vi "ConfigureIntake.vi"(10 "Talon In":T1) -> (2 "Talon Out":T1)   [LabVIEW 2018]
uses:
  <vilib>/Rock Robotics/WPI/MotorControl/WPI_MotorControlDeviceRef.ctl
  <vilib>/Rock Robotics/WPI/MotorControl/WPI_MotorControlType.ctl
  <vilib>/Rock Robotics/SystemInterfaces/DIO/FPGA_DIOPWMChannel.ctl
  <vilib>/Rock Robotics/WPI/PWM/WPI_PWMDeadband.ctl
  <vilib>/Rock Robotics/SystemInterfaces/DIO/FPGA_DIOChannel.ctl
  <vilib>/Rock Robotics/WPI/ThirdParty/Phoenix-LabVIEW/Motor Controller/Controls/CTRE_Phoenix_MotorControl_FeedbackDevice.ctl
  <vilib>/Rock Robotics/WPI/ThirdParty/Phoenix-LabVIEW/Motor Controller/Controls/CTRE_Phoenix_MotorControl_StatusFrameEnhanced.ctl
  <vilib>/Rock Robotics/WPI/ThirdParty/Phoenix-LabVIEW/Motor Controller/Controls/CTRE_Phoenix_MotorControl_NeutralMode.ctl
  <vilib>/Rock Robotics/WPI/ThirdParty/Phoenix-LabVIEW/Motor Controller/Controls/CTRE_Phoenix_MotorControl_ControlMode.ctl
  Intake Constants.vi
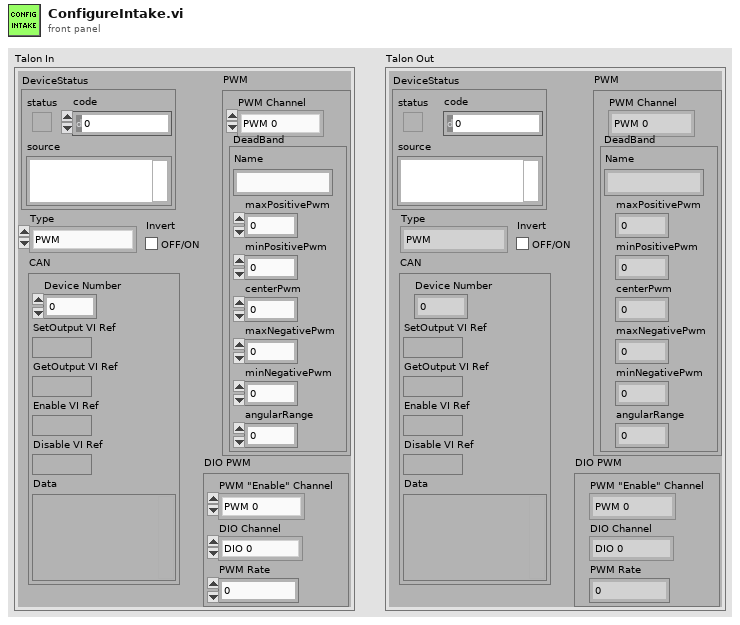
[diagram p1: front panel]
types:
  T1 = typedef "WPI_MotorControlDeviceRef.ctl" = cluster{"DeviceStatus":errorcluster, "Type":T2, "PWM":cluster{"PWM Channel":T3, "DeadBand":T4}, "CAN":cluster{"Device Number":u8, "SetOutput VI Ref":variant, "GetOutput VI Ref":variant, "Enable VI Ref":variant, "Disable VI Ref":variant, "Data":variant}, "Invert":bool, "DIO PWM":cluster{"PWM \"Enable\" Channel":T3, "DIOChannel":T5, "PWM Rate":dbl}}
  T2 = typedef "WPI_MotorControlType.ctl" = enum16{"PWM", "CAN", "DIO PWM"}
  T3 = typedef "FPGA_DIOPWMChannel.ctl" = enum8{"PWM 0", "PWM 1", "PWM 2", "PWM 3", "PWM 4", "PWM 5", "PWM 6", "PWM 7", "PWM 8", "PWM 9", "PWM MXP 0", "PWM MXP 1", "PWM MXP 2", "PWM MXP 3", "PWM MXP 4", "PWM MXP 5", "PWM MXP 6", "PWM MXP 7", "PWM MXP 8", "PWM MXP 9", "Invalid"}
  T4 = typedef "WPI_PWMDeadband.ctl" = cluster{"Name":string, "maxPositivePwm":i32, "minPositivePwm":i32, "centerPwm":i32, "maxNegativePwm":i32, "minNegativePwm":i32, "angularRange":u16}
  T5 = typedef "FPGA_DIOChannel.ctl" = enum8{"DIO 0", "DIO 1", "DIO 2", "DIO 3", "DIO 4", "DIO 5", "DIO 6", "DIO 7", "DIO 8", "DIO 9", "DIO MXP 0", "DIO MXP 1", "DIO MXP 2", "DIO MXP 3", "DIO MXP 4", "DIO MXP 5", "DIO MXP 6", "DIO MXP 7", "DIO MXP 8", "DIO MXP 9", "DIO MXP 10", "DIO MXP 11", "DIO MXP 12", "DIO MXP 13", "DIO MXP 14", "DIO MXP 15", "SPI Port CS1", "SPI Port CS2", "SPI Port CS3", "SPI Port MISO", "SPI Port MOSI", "Invalid"}
  T6 = typedef "CTRE_Phoenix_MotorControl_ControlMode.ctl" = u16
  T7 = typedef "CTRE_Phoenix_MotorControl_NeutralMode.ctl" = enum8{"EEPROMSetting", "Override to Coast", "Override to Brake"}
  T8 = typedef "CTRE_Phoenix_MotorControl_StatusFrameEnhanced.ctl" = u16
  T9 = typedef "CTRE_Phoenix_MotorControl_FeedbackDevice.ctl" = i8
  T10 = cluster{"kP":dbl, "kI ":dbl, "kD":dbl, "kF":dbl, "I Zone":dbl, "Peak Out":dbl}
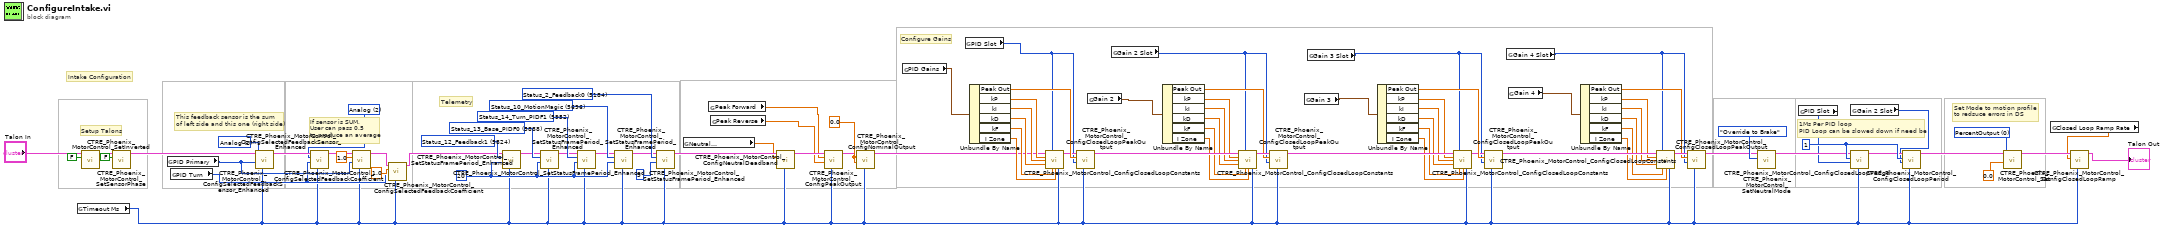
[diagram p0: block diagram]
diagram:
  w29 = T6 0 items=["PercentOutput"=0, "Position"=1, "Velocity"=2, "Current"=3, "Follower"=5, "MotionProfile"=6, "MotionMagic"=7, "MotionProfileArc"=10, "Disabled"=15] ("Control Mode")
  w87 = 1 ("loopTimeMs")
  w50 = 0.0 ("Forward Nominal Percent Output")
  w26 = 20 ("periodMs")
  w45 = T8 5184 items=["Status_1_General"=5120, "Status_2_Feedback0"=5184, "Status_3_Quadrature"=5248, "Status_4_AinTempVbat"=5312, "Status_6_Misc"=5440, "Status_7_CommStatus"=5504, "Status_8_PulseWidth"=5568, "Status_9_MotProfBuffer"=5632, "Status_10_MotionMagic"=5696, "Status_11_UartGadgeteer"=5760, "Status_12_Feedback1"=5824, "Status_13_Base_PIDF0"=5888, "Status_14_Turn_PIDF1"=5952, "Status_15_FirmwareApiStatus"=6016] ("Status Frame")
  w44 = T8 5696 items=["Status_1_General"=5120, "Status_2_Feedback0"=5184, "Status_3_Quadrature"=5248, "Status_4_AinTempVbat"=5312, "Status_6_Misc"=5440, "Status_7_CommStatus"=5504, "Status_8_PulseWidth"=5568, "Status_9_MotProfBuffer"=5632, "Status_10_MotionMagic"=5696, "Status_11_UartGadgeteer"=5760, "Status_12_Feedback1"=5824, "Status_13_Base_PIDF0"=5888, "Status_14_Turn_PIDF1"=5952, "Status_15_FirmwareApiStatus"=6016] ("Status Frame")
  w43 = T8 5952 items=["Status_1_General"=5120, "Status_2_Feedback0"=5184, "Status_3_Quadrature"=5248, "Status_4_AinTempVbat"=5312, "Status_6_Misc"=5440, "Status_7_CommStatus"=5504, "Status_8_PulseWidth"=5568, "Status_9_MotProfBuffer"=5632, "Status_10_MotionMagic"=5696, "Status_11_UartGadgeteer"=5760, "Status_12_Feedback1"=5824, "Status_13_Base_PIDF0"=5888, "Status_14_Turn_PIDF1"=5952, "Status_15_FirmwareApiStatus"=6016] ("Status Frame")
  w42 = T8 5888 items=["Status_1_General"=5120, "Status_2_Feedback0"=5184, "Status_3_Quadrature"=5248, "Status_4_AinTempVbat"=5312, "Status_6_Misc"=5440, "Status_7_CommStatus"=5504, "Status_8_PulseWidth"=5568, "Status_9_MotProfBuffer"=5632, "Status_10_MotionMagic"=5696, "Status_11_UartGadgeteer"=5760, "Status_12_Feedback1"=5824, "Status_13_Base_PIDF0"=5888, "Status_14_Turn_PIDF1"=5952, "Status_15_FirmwareApiStatus"=6016] ("Status Frame")
  w41 = T8 5824 items=["Status_1_General"=5120, "Status_2_Feedback0"=5184, "Status_3_Quadrature"=5248, "Status_4_AinTempVbat"=5312, "Status_6_Misc"=5440, "Status_7_CommStatus"=5504, "Status_8_PulseWidth"=5568, "Status_9_MotProfBuffer"=5632, "Status_10_MotionMagic"=5696, "Status_11_UartGadgeteer"=5760, "Status_12_Feedback1"=5824, "Status_13_Base_PIDF0"=5888, "Status_14_Turn_PIDF1"=5952, "Status_15_FirmwareApiStatus"=6016] ("Status Frame")
  w25 = T9 2 items=["None"=-1, "QuadEncoder"=0, "Analog"=2, "Tachometer"=4, "Pulse Width Encoded Position"=8, "Sensor Sum (S0 + S1)"=9, "Sensor Difference (D0 - D1)"=10, "Remote Source 0"=11, "Remote Source 1"=12, "Software Emulated"=15] ("Feedback Device")
  w33 = T9 2 items=["None"=-1, "QuadEncoder"=0, "Analog"=2, "Tachometer"=4, "Pulse Width Encoded Position"=8, "Sensor Sum (S0 + S1)"=9, "Sensor Difference (D0 - D1)"=10, "Remote Source 0"=11, "Remote Source 1"=12, "Software Emulated"=15] ("Feedback Device")
  # "Intake Configuration"
  # "Set Mode to motion profile\nto redsuce errors in DS"
  # "1Ms Per PID loop\nPID Loop can be slowed down if need be"
  # "Configure Gains"
  # "Setup Talons"
  # "Telemetry"
  # "If sensor is SUM,\nUser can pass 0.5\nto produce an average"
  # "This feedback sensor is the sum\nof left side and this one (right side)"
  n1 = global read "Intake Constants.vi" "Timeout Ms"() -> (w2:i32)
  n2 = call <vilib>:"CTRE_Phoenix_MotorControl_SetInverted.vi"("Invert?"=FALSE, "PhoenixMotorControlDevRef"="Talon In") -> ("PhoenixMotorControlDevRef"=w31:T1)  [unwired: 8 in, 1 out]
  n3 = call <vilib>:"CTRE_Phoenix_MotorControl_SetSensorPhase.vi"("PhaseSensor"=FALSE, "PhoenixMotorControlDevRef"=w31) -> ("PhoenixMotorControlDevRef"=w22:T1)  [unwired: 8 in, 1 out]
  n4 = global read "Intake Constants.vi" "PID Primary"() -> (w19:i32)
  n5 = global read "Intake Constants.vi" "PID Turn"() -> (w18:i32)
  n6 = call <vilib>:"CTRE_Phoenix_MotorControl_ConfigSelectedFeedbackSensor_Enhanced.vi"("timeoutMs"=w2, "pidLoopIdx"=w19, "Feedback Device"=w33, "PhoenixMotorControlDevRef"=w22) -> ("PhoenixMotorControlDevRef"=w34:T1)  [unwired: 6 in, 1 out]
  n7 = call <vilib>:"CTRE_Phoenix_MotorControl_ConfigSelectedFeedbackSensor_Enhanced.vi"("timeoutMs"=w2, "pidLoopIdx"=w18, "Feedback Device"=w25, "PhoenixMotorControlDevRef"=w34) -> ("PhoenixMotorControlDevRef"=w35:T1)  [unwired: 6 in, 1 out]
  n8 = call <vilib>:"CTRE_Phoenix_MotorControl_ConfigSelectedFeedbackCoefficient.vi"("timoutMs"=w2, "pidIdx"=w19, "coefficient"=1.0, "PhoenixMotorControlDevRef"=w35) -> ("PhoenixMotorControlDevRef"=w24:T1)  [unwired: 6 in, 1 out]
  n9 = call <vilib>:"CTRE_Phoenix_MotorControl_ConfigSelectedFeedbackCoefficient.vi"("timoutMs"=w2, "pidIdx"=w18, "coefficient"=1.0, "PhoenixMotorControlDevRef"=w24) -> ("PhoenixMotorControlDevRef"=w23:T1)  [unwired: 6 in, 1 out]
  n10 = call <vilib>:"CTRE_Phoenix_MotorControl_SetStatusFramePeriod_Enhanced.vi"("timeoutMs"=w2, "periodMs"=w26, "Status Frame"=w41, "PhoenixMotorControlDevRef"=w23) -> ("PhoenixMotorControlDevRef"=w37:T1)  [unwired: 6 in, 1 out]
  n11 = call <vilib>:"CTRE_Phoenix_MotorControl_SetStatusFramePeriod_Enhanced.vi"("timeoutMs"=w2, "periodMs"=w26, "Status Frame"=w42, "PhoenixMotorControlDevRef"=w37) -> ("PhoenixMotorControlDevRef"=w38:T1)  [unwired: 6 in, 1 out]
  n12 = call <vilib>:"CTRE_Phoenix_MotorControl_SetStatusFramePeriod_Enhanced.vi"("timeoutMs"=w2, "periodMs"=w26, "Status Frame"=w43, "PhoenixMotorControlDevRef"=w38) -> ("PhoenixMotorControlDevRef"=w39:T1)  [unwired: 6 in, 1 out]
  n13 = call <vilib>:"CTRE_Phoenix_MotorControl_SetStatusFramePeriod_Enhanced.vi"("timeoutMs"=w2, "periodMs"=w26, "Status Frame"=w44, "PhoenixMotorControlDevRef"=w39) -> ("PhoenixMotorControlDevRef"=w40:T1)  [unwired: 6 in, 1 out]
  n14 = call <vilib>:"CTRE_Phoenix_MotorControl_SetStatusFramePeriod_Enhanced.vi"("timeoutMs"=w2, "periodMs"=5, "Status Frame"=w45, "PhoenixMotorControlDevRef"=w40) -> ("PhoenixMotorControlDevRef"=w47:T1)  [unwired: 6 in, 1 out]
  n15 = global read "Intake Constants.vi" "Neutral\nDeadband"() -> (w17:dbl)
  n16 = global read "Intake Constants.vi" "Peak Forward"() -> (w16:dbl)
  n17 = global read "Intake Constants.vi" "Peak Reverse"() -> (w15:dbl)
  n18 = call <vilib>:"CTRE_Phoenix_MotorControl_ConfigNeutralDeadband.vi"("timeoutMs"=w2, "Percent Deadband"=w17, "PhoenixMotorControlDevRef"=w47) -> ("PhoenixMotorControlDevRef"=w48:T1)  [unwired: 7 in, 1 out]
  n19 = call <vilib>:"CTRE_Phoenix_MotorControl_ConfigPeakOutput.vi"("timeoutMs"=w2, "Reverse Peak Percent Output"=w15, "Forward Peak Percent Output"=w16, "PhoenixMotorControlDevRef"=w48) -> ("PhoenixMotorControlDevRef"=w49:T1)  [unwired: 6 in, 1 out]
  n20 = call <vilib>:"CTRE_Phoenix_MotorControl_ConfigNominalOutput.vi"("timeoutMs"=w2, "Reverse Nominal Percent Output"=w50, "Forward Nominal Percent Output"=w50, "PhoenixMotorControlDevRef"=w49) -> ("PhoenixMotorControlDevRef"=w51:T1)  [unwired: 6 in, 1 out]
  n21 = global read "Intake Constants.vi" "PID Gains"() -> (w14:T10)
  n22 = global read "Intake Constants.vi" "PID Slot"() -> (w13:i32)
  n23 = Unbundle By Name(w14) -> ("Peak Out"=w58:dbl, "kP"=w52:dbl, "kI"=w53:dbl, "kD"=w54:dbl, "kF"=w55:dbl, "I Zone"=w56:dbl)
  n24 = call <vilib>:"CTRE_Phoenix_MotorControl_ConfigClosedLoopConstants.vi"("PhoenixMotorControlDevRef"=w51, "slotIdx"=w13, "P"=w52, "I"=w53, "D"=w54, "F"=w55, "I Zone"=w56, "timeoutMs"=w2) -> ("PhoenixMotorControlDevRef"=w57:T1)  [unwired: 6 in, 1 out]
  n25 = call <vilib>:"CTRE_Phoenix_MotorControl_ConfigClosedLoopPeakOutput.vi"("timoutMs"=w2, "slotIdx"=w13, "peakOutput"=w58, "PhoenixMotorControlDevRef"=w57) -> ("PhoenixMotorControlDevRef"=w80:T1)  [unwired: 6 in, 1 out]
  n26 = global read "Intake Constants.vi" "Gain 2"() -> (w12:T10)
  n27 = global read "Intake Constants.vi" "Gain 2 Slot"() -> (w11:i32)
  n28 = Unbundle By Name(w12) -> ("Peak Out"=w59:dbl, "kP"=w65:dbl, "kI"=w64:dbl, "kD"=w63:dbl, "kF"=w62:dbl, "I Zone"=w61:dbl)
  n29 = call <vilib>:"CTRE_Phoenix_MotorControl_ConfigClosedLoopConstants.vi"("PhoenixMotorControlDevRef"=w80, "slotIdx"=w11, "P"=w65, "I"=w64, "D"=w63, "F"=w62, "I Zone"=w61, "timeoutMs"=w2) -> ("PhoenixMotorControlDevRef"=w60:T1)  [unwired: 6 in, 1 out]
  n30 = call <vilib>:"CTRE_Phoenix_MotorControl_ConfigClosedLoopPeakOutput.vi"("timoutMs"=w2, "slotIdx"=w11, "peakOutput"=w59, "PhoenixMotorControlDevRef"=w60) -> ("PhoenixMotorControlDevRef"=w81:T1)  [unwired: 6 in, 1 out]
  n31 = global read "Intake Constants.vi" "Gain 3"() -> (w10:T10)
  n32 = global read "Intake Constants.vi" "Gain 3 Slot"() -> (w9:i32)
  n33 = Unbundle By Name(w10) -> ("Peak Out"=w72:dbl, "kP"=w66:dbl, "kI"=w67:dbl, "kD"=w68:dbl, "kF"=w69:dbl, "I Zone"=w70:dbl)
  n34 = call <vilib>:"CTRE_Phoenix_MotorControl_ConfigClosedLoopConstants.vi"("PhoenixMotorControlDevRef"=w81, "slotIdx"=w9, "P"=w66, "I"=w67, "D"=w68, "F"=w69, "I Zone"=w70, "timeoutMs"=w2) -> ("PhoenixMotorControlDevRef"=w71:T1)  [unwired: 6 in, 1 out]
  n35 = call <vilib>:"CTRE_Phoenix_MotorControl_ConfigClosedLoopPeakOutput.vi"("timoutMs"=w2, "slotIdx"=w9, "peakOutput"=w72, "PhoenixMotorControlDevRef"=w71) -> ("PhoenixMotorControlDevRef"=w82:T1)  [unwired: 6 in, 1 out]
  n36 = global read "Intake Constants.vi" "Gain 4 Slot"() -> (w7:i32)
  n37 = global read "Intake Constants.vi" "Gain 4"() -> (w8:T10)
  n38 = Unbundle By Name(w8) -> ("Peak Out"=w73:dbl, "kP"=w79:dbl, "kI"=w78:dbl, "kD"=w77:dbl, "kF"=w76:dbl, "I Zone"=w75:dbl)
  n39 = call <vilib>:"CTRE_Phoenix_MotorControl_ConfigClosedLoopConstants.vi"("PhoenixMotorControlDevRef"=w82, "slotIdx"=w7, "P"=w79, "I"=w78, "D"=w77, "F"=w76, "I Zone"=w75, "timeoutMs"=w2) -> ("PhoenixMotorControlDevRef"=w74:T1)  [unwired: 6 in, 1 out]
  n40 = call <vilib>:"CTRE_Phoenix_MotorControl_ConfigClosedLoopPeakOutput.vi"("timoutMs"=w2, "slotIdx"=w7, "peakOutput"=w73, "PhoenixMotorControlDevRef"=w74) -> ("PhoenixMotorControlDevRef"=w83:T1)  [unwired: 6 in, 1 out]
  n41 = call <vilib>:"CTRE_Phoenix_MotorControl_SetNeutralMode.vi"("Motor Control Neutral Mode"=CTRE_Phoenix_MotorControl_NeutralMode."Override to Brake", "PhoenixMotorControlDevRef"=w83) -> ("PhoenixMotorControlDevRef"=w85:T1)  [unwired: 8 in, 1 out]
  n42 = global read "Intake Constants.vi" "PID Slot"() -> (w5:i32)
  n43 = global read "Intake Constants.vi" "Gain 2 Slot"() -> (w6:i32)
  n44 = call <vilib>:"CTRE_Phoenix_MotorControl_ConfigClosedLoopPeriod.vi"("timoutMs"=w2, "slotIdx"=w5, "loopTimeMs"=w87, "PhoenixMotorControlDevRef"=w85) -> ("PhoenixMotorControlDevRef"=w86:T1)  [unwired: 6 in, 1 out]
  n45 = call <vilib>:"CTRE_Phoenix_MotorControl_ConfigClosedLoopPeriod.vi"("timoutMs"=w2, "slotIdx"=w6, "loopTimeMs"=w87, "PhoenixMotorControlDevRef"=w86) -> ("PhoenixMotorControlDevRef"=w20:T1)  [unwired: 6 in, 1 out]
  n46 = call <vilib>:"CTRE_Phoenix_MotorControl_Set.vi"("Output"=0.0, "Control Mode"=w29, "PhoenixMotorControlDevRef"=w20) -> ("PhoenixMotorControlDevRef"=w4:T1)  [unwired: 7 in, 1 out]
  n47 = global read "Intake Constants.vi" "Closed Loop Ramp Rate"() -> (w1:dbl)
  n48 = call <vilib>:"CTRE_Phoenix_MotorControl_ConfigClosedLoopRamp.vi"("timeoutMs"=w2, "secondsFromNeutralToFull"=w1, "PhoenixMotorControlDevRef"=w4) -> ("PhoenixMotorControlDevRef"=→"Talon Out":T1)  [unwired: 7 in, 1 out]
